vi "RemoteControl.SendMessageFromProcess.vi"(8 "error in (no error)":errorcluster, 10 "Message":T1, 11 "RemoteControl":refnum<class "RemoteControl.lvclass">) -> (0 "error out":errorcluster, 3 "RemoteControl out":refnum<class "RemoteControl.lvclass">)   [LabVIEW 2019, in "RemoteControl.lvclass"]
doc: "---------------------------------------------------------------\nJKI State Machine Objects™\nhttp://jki.net/state-machine-objects/\nCopyright (C) 2005-2015, JKI <info@jki.net>\nALL RIGHTS RESERVEDJKI State Machine Objects (SMO) 1.0.0.4\nJKI - JKI\nCopyright (c) 2015, JKI"
uses:
  RemoteControl.lvclass
  Typedefs/Message--Cluster.ctl
  RemoteControl.lvclass/RemoteControl.ctl
  Typedefs/PublicEvents--RemoteControl.SendMessageFromProcess.ctl
panel:
  # "For instructions on how to use the JKI State Machine Objects, examples and video tutorials, visit:\nhttp://jki.net/state-machine-objects/\n\nJKI State Machine Objects™\nhttp://jki.net/state-machine-objects/\nCopyright (C) 2005-2015, JKI <info@jki.net>\nALL RIGHTS RESERVED"
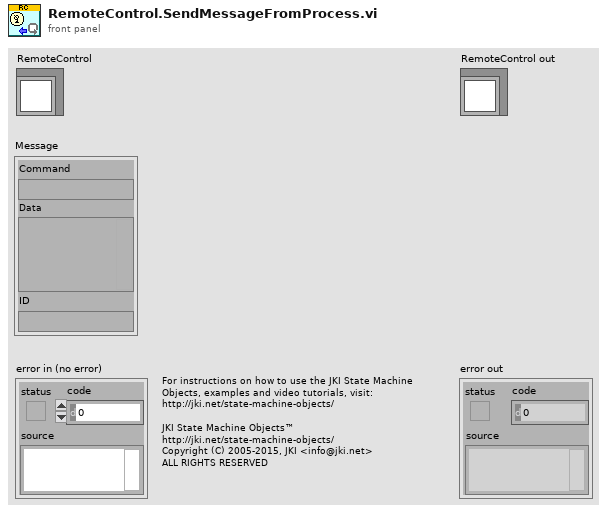
[diagram p1: front panel]
types:
  T1 = typedef "RemoteControl.lvclass/Message--Cluster.ctl" = cluster{"Command":string, "Data":variant, "ID":string}
  T2 = typedef "RemoteControl.lvclass/PublicEvents--RemoteControl.SendMessageFromProcess.ctl" = cluster{"Message":T1}
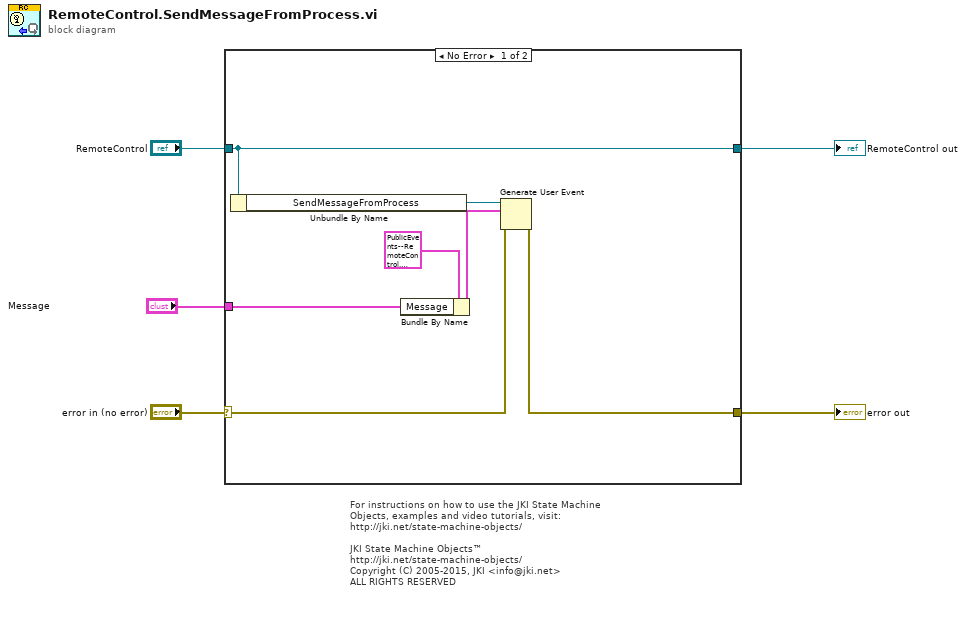
[diagram p0: block diagram]
diagram:
  # "For instructions on how to use the JKI State Machine Objects, examples and video tutorials, visit:\nhttp://jki.net/state-machine-objects/\n\nJKI State Machine Objects™\nhttp://jki.net/state-machine-objects/\nCopyright (C) 2005-2015, JKI <info@jki.net>\nALL RIGHTS RESERVED"
  n1 = case shown="No Error" "error in (no error)" {
    selector: "error in (no error)" -> [w12 w14]
    tunnel: [w10 w14] -> w4
    tunnel: [w9 w13] -> w5
    tunnel: "RemoteControl" -> [w9 w13]
    tunnel: "Message" -> [w7 _]
    frame No Error {
      n2 = Unbundle By Name(w9) -> ("SendMessageFromProcess"=w11:refnum<user-event>)
      n3 = Bundle By Name(cluster=T2 {"Message"={"Command"="", "Data"=variant(string ""), "ID"=""}} ("SendMessageFromProcess"), "Message"=w7) -> (w6:T2)
      n4 = Generate User Event(user event=w11, event data cluster=w6, error in=w12) -> (error out=w10:errorcluster)  [unwired: 1 in, 1 out]
    }
    frame Error {
    }
  }
  "error out" <- w4
  "RemoteControl out" <- w5
